vi "runscenario export Results.vi"(8 "error in (no error)":errorcluster, 9 "POST (empty)":T1, 10 "GET Parameter (\"\")":string) -> (0 "error out":errorcluster, 1 "Filename":string, 2 "Content":string)   [LabVIEW 2011]
uses:
  Addons/internet/utils/keyedarr.llb/Keyed Array.ctl
  Addons/internet/utils/strutil.llb/Case Matching.ctl
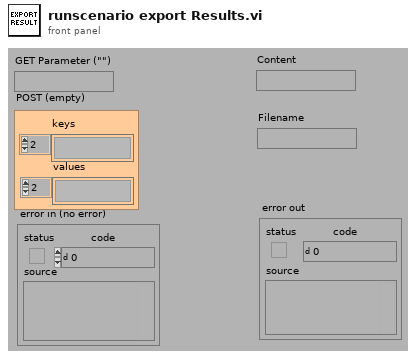
[diagram p1: front panel]
types:
  T1 = typedef "Keyed Array.ctl" = cluster{"keys":string[], "values":string[]}
  T2 = typedef "Case Matching.ctl" = enum16{"a != A", "a == A", "system"}
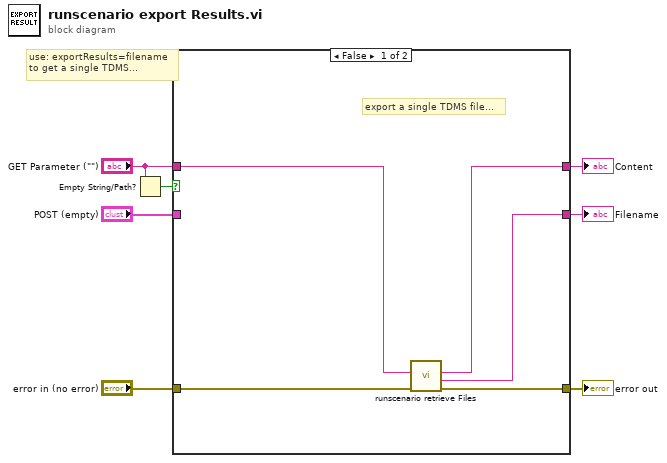
[diagram p0: block diagram]
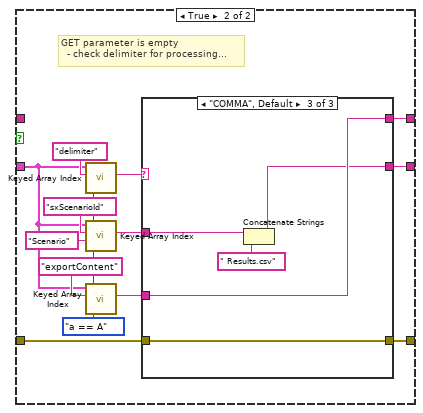
[diagram p2: hidden frame]
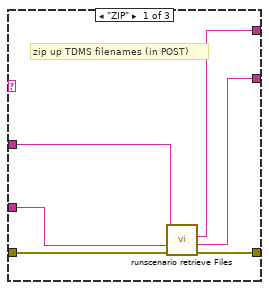
[diagram p3: hidden frame]
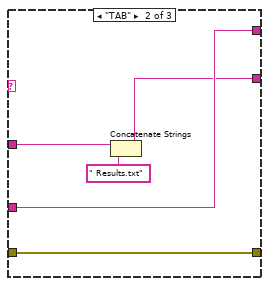
[diagram p4: hidden frame]
diagram:
  # "use: exportResults=filename\nto get a single TDMS..."
  n1 = Empty String/Path?(string/path="GET Parameter (\"\")") -> (empty?=w5:bool)
  n2 = case shown="False" w5 {
    tunnel: "error in (no error)" -> [w12 w25]
    tunnel: [w11 w24] -> w6
    tunnel: "GET Parameter (\"\")" -> [w10 _]
    tunnel: [w9 w22] -> w3
    tunnel: [w8 w21] -> w2
    tunnel: "POST (empty)" -> [_ w14]
    frame False {
      # "export a single TDMS file..."
      n3 = call "runscenario retrieve Files.vi"("error in (no error)"=w12, "filename (\"\": use POST)"=w10) -> ("error out"=w11:errorcluster, "Filename"=w8:string, "Content"=w9:string)  [unwired: 3 in, 4 out]
    }
    frame True {
      w15 = Case_Matching."a == A" ("case matching (sensitive)")
      # "GET parameter is empty\n  - check delimiter for processing..."
      n4 = call "Keyed Array Index.vi"("case matching (sensitive)"=w15, "key"="delimiter" ("Template (\"\")"), "array in"=w14) -> ("value"=w20:string)  [unwired: 1 in, 3 out]
      n5 = call "Keyed Array Index.vi"("case matching (sensitive)"=w15, "default value"="Scenario" ("key"), "key"="sxScenarioId", "array in"=w14) -> ("value"=w13:string)  [unwired: 3 out]
      n6 = call "Keyed Array Index.vi"("case matching (sensitive)"=w15, "key"="exportContent" ("Template (\"\")"), "array in"=w14) -> ("value"=w18:string)  [unwired: 1 in, 3 out]
      n7 = case shown="\"COMMA\", Default" w20 {
        tunnel: w25 -> [w31 w36 w41]
        tunnel: [w30 w36 w41] -> w24
        tunnel: [w28 w35 w40] -> w22
        tunnel: [w29 w32 w37] -> w21
        tunnel: w18 -> [w27 w35 w40]
        tunnel: w13 -> [w26 w34 w39]
        frame "ZIP" {
          # "zip up TDMS filenames (in POST)"
          n8 = call "runscenario retrieve Files.vi"("error in (no error)"=w31, "exportContent (\"\")"=w27, "sxScenarioId (\"\")"=w26) -> ("error out"=w30:errorcluster, "Filename"=w29:string, "Content"=w28:string)  [unwired: 2 in, 4 out]
        }
        frame "TAB" {
          n9 = Concatenate Strings(w34, " Results.txt" ("Template (\"\")")) -> (w32:string)
        }
        frame "COMMA", Default {
          n10 = Concatenate Strings(w39, " Results.csv" ("Template (\"\")")) -> (w37:string)
        }
      }
    }
  }
  "error out" <- w6
  "Content" <- w3
  "Filename" <- w2
